vi "Check for Fresh Message.vi"(8 "error in":errorcluster, 11 "Handle Chirp Request in":refnum<class "Handle Chirp Request.lvclass">) -> (0 "error out":errorcluster, 1 "Enqueuer":refnum<class "Message Enqueuer.lvclass">, 2 "Enqueuer not Valid":bool, 3 "Handle Chirp Request out":refnum<class "Handle Chirp Request.lvclass">)   [LabVIEW 2014, in "Handle Chirp Request.lvclass"]
doc: "This method is a dynamic method that \n1) checks for a good connection to the shared variable. If it is not present, then it attempts to connect If a connection is not available, then this VI will do nothing.\n2) Check the state of the enqueuer. If the state is no good, return with this indication and do nothing.\n2) If the connection is good, check to see if the current shared variable state has changed.\n3) If the state has changed, pump the message into the appropriate enqueuer."
uses:
  Handle Chirp Request.lvclass
  <vilib>/ActorFramework/Message Enqueuer/Message Enqueuer.lvclass
  Instr Actor/Messages/Change Speaker Chirp/Send New Chirp MSG.lvclass
  Instr Actor/Messages/Change Speaker Chirp/Send New Chirp MSG.lvclass/Send New Chirp MSG.ctl
  <vilib>/ActorFramework/Message Enqueuer/Message Enqueuer.lvclass/Message Enqueuer.ctl
  Instr Actor/Messages/Change Speaker Chirp/Write f0.vi
  Instr Actor/Messages/Change Speaker Chirp/Write Df.vi
  <vilib>/ActorFramework/Message Priority Queue/Priority Enqueue.vi
  Network Command Processor.lvclass
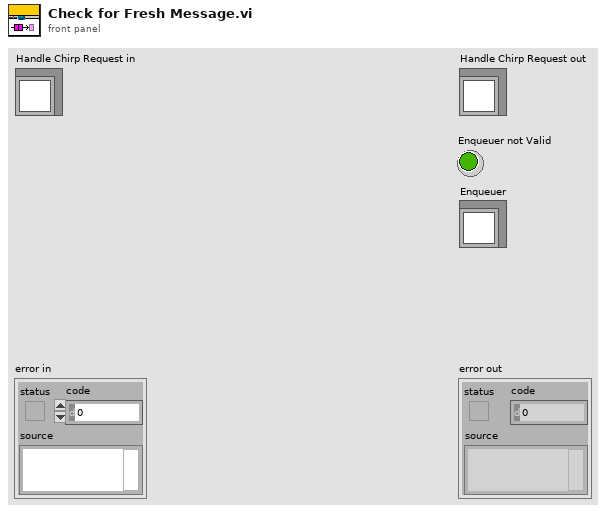
[diagram p1: front panel]
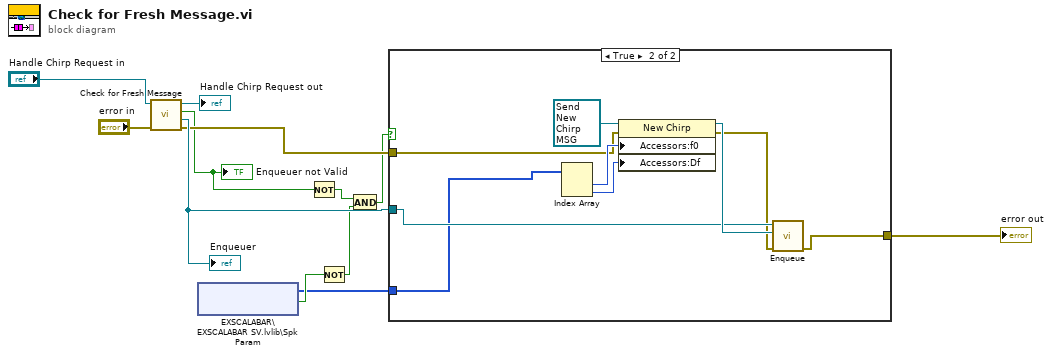
[diagram p0: block diagram]
diagram:
  n1 = call-parent "Check for Fresh Message.vi"("error in"="error in", "Network Command Processor in"="Handle Chirp Request in") -> ("error out"=w8:errorcluster, "Enqueuer"=w9:refnum<class "Message Enqueuer.lvclass">, "Enqueuer not Valid"=w5:bool, "Network Command Processor out"=→"Handle Chirp Request out":refnum<class "Handle Chirp Request.lvclass">)  [unwired: 6 in]
  "Enqueuer not Valid" <- w5
  "Enqueuer" <- w9
  n2 = shared-variable "EXSCALABAR\\EXSCALABAR SV.lvlib\\Spk Param"() -> (w1:i16[], w6:bool)  [unwired: 2 in, 1 out]
  n3 = Not(x=w5) -> (.not. x?=w4:bool)
  n4 = Not(x=w6) -> (.not. x?=w3:bool)
  n5 = And(x=w4, y=w3) -> (x .and. y?=w2:bool)
  n6 = case shown="True" w2 {
    tunnel: w9 -> [_ w17]
    tunnel: w8 -> [_ w15]
    tunnel: [_ w14] -> w7
    tunnel: w1 -> [_ w13]
    frame False {
    }
    frame True {
      n7 = Index Array(array=w13) -> (element #1=w20:i16, element #2=w21:i16)  [unwired: 2 in]
      n8 = property class="New Chirp"(reference=refnum<class "Send New Chirp MSG.lvclass"> refnum ("Instrument Lib:New Chirp"), error in=w15, "Accessors:f0"=w20, "Accessors:Df"=w21) -> (reference out=w18:refnum<class "Send New Chirp MSG.lvclass">, error out=w16:errorcluster)
      n9 = call <vilib>:"Enqueue.vi"("error in (no error)"=w16, "Message"=w18, "Message Enqueuer in"=w17) -> ("error out"=w14:errorcluster)  [unwired: 7 in, 1 out]
    }
  }
  "error out" <- w7
